vi "Visa Write Trigger.vi"() -> ()   [LabVIEW 2022 SP3]
uses:
  <vilib>/Instr/_visa.llb/Select Event Type.ctl
panel:
  in  "2400 CURR LIST":string="20E-6,-20E-6"
  out "Resistance of DUT":dbl[](graph)
  out "Resistance (m-Ohms)":dbl[](array[numeric]) format="%.10f"
  in  "Sample Count To Display":i32=10
  out "Voltage Drop Across DUT":dbl[](graph)
  out "Delta Readings (uV)":ext[](array[numeric]) format="%.12f"
  in  "2400 Trig Count":string="20"
  in  "2182A":T1={"Baud Rate"=9600, "Parity"=0, "Data Bits"=8, "Stop Bits"=10, "Flow Control"=0, "VISA resource name"="NanoVoltMeter2182"} {"Flow Control" items=["None", "XON/XOFF", "RTS/CTS", "XON/XOFF & RTS/CTS", "DTR/DSR", "XON/XOFF & DTR/DSR"]; "Stop Bits" items=["1.0"=10, "1.5"=15, "2.0"=20]; "Data Bits" items=["7"=7, "8"=8]; "Parity" items=["None", "Odd", "Even", "Mark", "Space"]; "Baud Rate" items=["300"=300, "600"=600, "1200"=1200, "2400"=2400, "4800"=4800, "9600"=9600, "19200"=19200]}
  in  "2400":T1={"Baud Rate"=9600, "Parity"=0, "Data Bits"=8, "Stop Bits"=10, "Flow Control"=0, "VISA resource name"="NanoVoltMeter2182"} {"Flow Control" items=["None", "XON/XOFF", "RTS/CTS", "XON/XOFF & RTS/CTS", "DTR/DSR", "XON/XOFF & DTR/DSR"]; "Stop Bits" items=["1.0"=10, "1.5"=15, "2.0"=20]; "Data Bits" items=["7"=7, "8"=8]; "Parity" items=["None", "Odd", "Even", "Mark", "Space"]; "Baud Rate" items=["300"=300, "600"=600, "1200"=1200, "2400"=2400, "4800"=4800, "9600"=9600, "19200"=19200]}
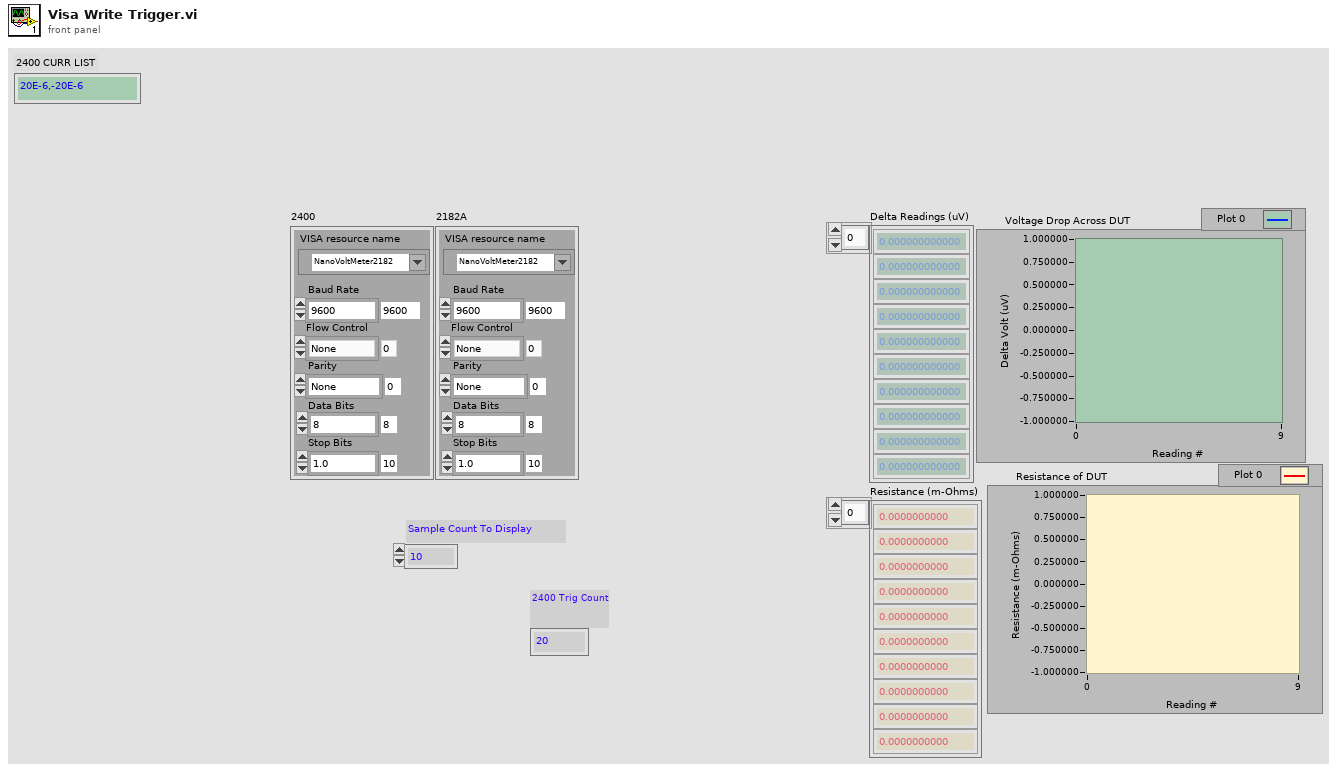
[diagram p1: front panel]
types:
  T1 = cluster{"Baud Rate":u32, "Parity":u16, "Data Bits":u16, "Stop Bits":u16, "Flow Control":u16, "VISA resource name":refnum<visa-resource-name>}
  T2 = typedef "Select Event Type.ctl" = u32
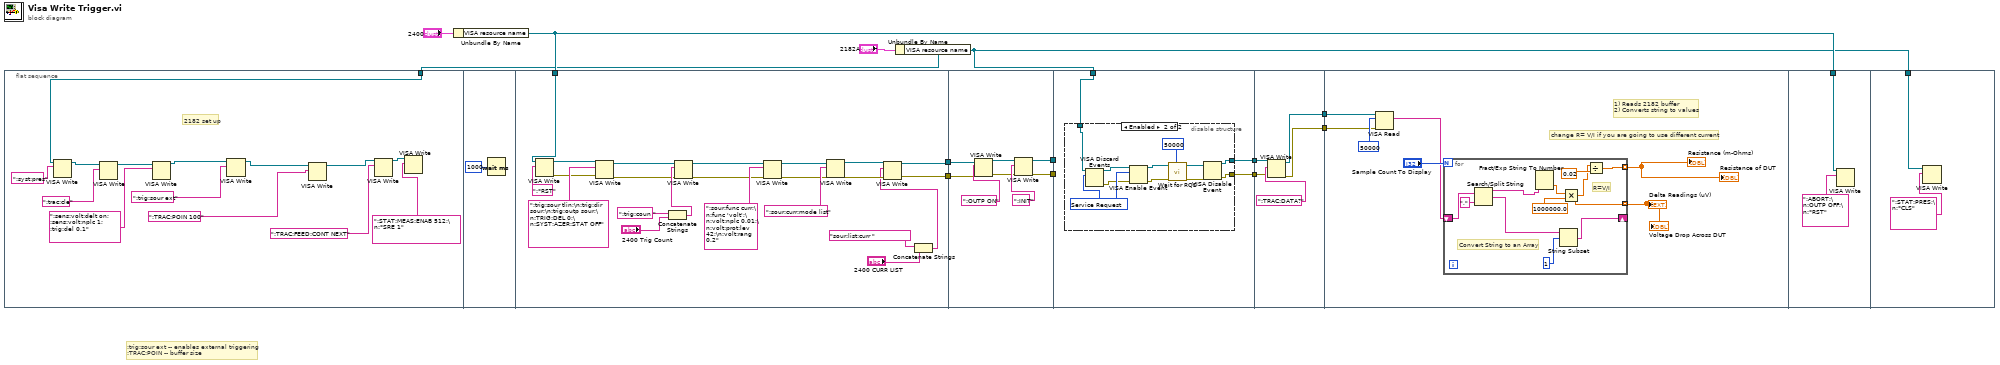
[diagram p0: block diagram]
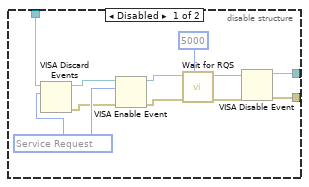
[diagram p2: hidden frame]
diagram:
  # ":trig:sour ext -- enables external triggering\n:TRAC:POIN -- buffer size"
  n1 = flat-sequence {
    tunnel: w2 -> [w25]
    tunnel: w6 -> [w50]
    tunnel: [w33] -> w11
    tunnel: [w32] -> w1
    tunnel: w11 -> [w58]
    tunnel: [w52] -> w10
    tunnel: [w51] -> w9
    tunnel: w1 -> [w54]
    tunnel: w10 -> [_]
    tunnel: w9 -> [_]
    tunnel: w2 -> [w61]
    tunnel: [w60] -> w5
    tunnel: [w59] -> w4
    tunnel: [w87] -> w8
    tunnel: [w86] -> w7
    tunnel: w5 -> [w85]
    tunnel: w4 -> [w84]
    tunnel: w8 -> [w90]
    tunnel: w7 -> [w89]
    tunnel: w6 -> [w108]
    tunnel: w2 -> [w110]
    frame #0 {
      # "2182 set up"
      n2 = VISA Write(VISA resource name=w25, write buffer=":syst:pres") -> (VISA resource name out=w24:refnum<visa-resource-name>)  [unwired: 1 in, 2 out]
      n3 = VISA Write(VISA resource name=w24, write buffer=":trac:cle") -> (VISA resource name out=w23:refnum<visa-resource-name>)  [unwired: 1 in, 2 out]
      n4 = VISA Write(VISA resource name=w23, write buffer=":sens:volt:delt on; :sens:volt:nplc 1; :trig:del 0.1") -> (VISA resource name out=w22:refnum<visa-resource-name>)  [unwired: 1 in, 2 out]
      n5 = VISA Write(VISA resource name=w22, write buffer=":trig:sour ext") -> (VISA resource name out=w21:refnum<visa-resource-name>)  [unwired: 1 in, 2 out]
      n6 = VISA Write(VISA resource name=w21, write buffer=":TRAC:POIN 100") -> (VISA resource name out=w20:refnum<visa-resource-name>)  [unwired: 1 in, 2 out]
      n7 = VISA Write(VISA resource name=w20, write buffer=":TRAC:FEED:CONT NEXT") -> (VISA resource name out=w19:refnum<visa-resource-name>)  [unwired: 1 in, 2 out]
      n8 = VISA Write(VISA resource name=w19, write buffer=":STAT:MEAS:ENAB 512;\n:*SRE 1") -> ()  [unwired: 1 in, 3 out]
    }
    frame #1 {
      n9 = Wait (ms)(milliseconds to wait=u32 1000) -> ()  [unwired: 1 out]
    }
    frame #2 {
      n10 = VISA Write(VISA resource name=w50, write buffer=":*RST") -> (VISA resource name out=w48:refnum<visa-resource-name>, error out=w38:errorcluster)  [unwired: 1 in, 1 out]
      n11 = VISA Write(VISA resource name=w48, write buffer=":trig:sour tlin;\n:trig:dir sour;\n:trig:outp sour;\n:TRIG:DEL 0;\n:SYST:AZER:STAT OFF", error in (no error)=w38) -> (VISA resource name out=w47:refnum<visa-resource-name>, error out=w37:errorcluster)  [unwired: 1 out]
      n12 = Concatenate Strings(":trig:coun ", "2400 Trig Count") -> (w41:string)
      n13 = VISA Write(VISA resource name=w47, write buffer=w41, error in (no error)=w37) -> (VISA resource name out=w46:refnum<visa-resource-name>, error out=w36:errorcluster)  [unwired: 1 out]
      n14 = VISA Write(VISA resource name=w46, write buffer=":sour:func curr;\n:func 'volt';\n:volt:nplc 0.01;\n:volt:prot:lev 42;\n:volt:rang 0.2", error in (no error)=w36) -> (VISA resource name out=w45:refnum<visa-resource-name>, error out=w35:errorcluster)  [unwired: 1 out]
      n15 = VISA Write(VISA resource name=w45, write buffer=":sour:curr:mode list", error in (no error)=w35) -> (VISA resource name out=w34:refnum<visa-resource-name>, error out=w31:errorcluster)  [unwired: 1 out]
      n16 = Concatenate Strings("sour:list:curr ", "2400 CURR LIST") -> (w28:string)
      n17 = VISA Write(VISA resource name=w34, write buffer=w28, error in (no error)=w31) -> (VISA resource name out=w33:refnum<visa-resource-name>, error out=w32:errorcluster)  [unwired: 1 out]
    }
    frame #3 {
      n18 = VISA Write(VISA resource name=w58, write buffer=":OUTP ON", error in (no error)=w54) -> (VISA resource name out=w57:refnum<visa-resource-name>, error out=w53:errorcluster)  [unwired: 1 out]
      n19 = VISA Write(VISA resource name=w57, write buffer=":INIT", error in (no error)=w53) -> (VISA resource name out=w52:refnum<visa-resource-name>, error out=w51:errorcluster)  [unwired: 1 out]
    }
    frame #4 {
      n20 = disable-structure shown="Enabled" {
        disable-tunnel: w61 -> [w71 w75]
        disable-tunnel: [w64 w74] -> w60
        disable-tunnel: [w62 w73] -> w59
        frame Disabled {
          w68 = T2 1073684491 items=["Service Request"=1073684491, "Trigger"=3221168138, "Clear"=1073684493, "VXI Signal"=1073684512, "VXI/VME Interrupt"=3221168161, "VXI/VME Sysfail"=1073684509, "VXI/VME Sysreset"=1073684510, "GPIB CIC"=1073684498, "GPIB Talk"=1073684499, "GPIB Listen"=1073684500, "PXI Interrupt"=1073684514, "Serial Break"=1073684515, "Serial TermChar"=1073684516, "Serial CTS"=1073684521, "Serial DSR"=1073684522, "Serial DCD"=1073684524, "Serial RI"=1073684526, "Serial Character"=1073684533, "USB Interrupt"=1073684535, "All Enabled"=1073709055] ("Event Type")
          n21 = VISA Discard Events(10:w68, 11:w71) -> (0:w66:errorcluster, 3:w70:refnum<visa-resource-name>)  [unwired: 2 in]
          n22 = VISA Enable Event(8:w66, 10:w68, 11:w70) -> (0:w67:errorcluster, 3:w69:refnum<visa-resource-name>)  [unwired: 1 in]
          n23 = call <vilib>:"Wait for RQS.vi"("timeout (25000 ms)"=u32 5000, "error in (no error)"=w67, "VISA resource name"=w69) -> ("error out"=w63:errorcluster, "VISA resource name out"=w65:refnum<visa-resource-name>)  [unwired: 6 in, 1 out]
          n24 = VISA Disable Event(8:w63, 11:w65) -> (0:w62:errorcluster, 3:w64:refnum<visa-resource-name>)  [unwired: 2 in]
        }
        frame Enabled {
          w80 = T2 1073684491 items=["Service Request"=1073684491, "Trigger"=3221168138, "Clear"=1073684493, "VXI Signal"=1073684512, "VXI/VME Interrupt"=3221168161, "VXI/VME Sysfail"=1073684509, "VXI/VME Sysreset"=1073684510, "GPIB CIC"=1073684498, "GPIB Talk"=1073684499, "GPIB Listen"=1073684500, "PXI Interrupt"=1073684514, "Serial Break"=1073684515, "Serial TermChar"=1073684516, "Serial CTS"=1073684521, "Serial DSR"=1073684522, "Serial DCD"=1073684524, "Serial RI"=1073684526, "Serial Character"=1073684533, "USB Interrupt"=1073684535, "All Enabled"=1073709055] ("Event Type")
          n25 = VISA Discard Events(10:w80, 11:w75) -> (0:w78:errorcluster, 3:w82:refnum<visa-resource-name>)  [unwired: 2 in]
          n26 = VISA Enable Event(8:w78, 10:w80, 11:w82) -> (0:w79:errorcluster, 3:w81:refnum<visa-resource-name>)  [unwired: 1 in]
          n27 = call <vilib>:"Wait for RQS.vi"("timeout (25000 ms)"=u32 50000, "error in (no error)"=w79, "VISA resource name"=w81) -> ("error out"=w76:errorcluster, "VISA resource name out"=w77:refnum<visa-resource-name>)  [unwired: 6 in, 1 out]
          n28 = VISA Disable Event(8:w76, 11:w77) -> (0:w73:errorcluster, 3:w74:refnum<visa-resource-name>)  [unwired: 2 in]
        }
      }
    }
    frame #5 {
      n29 = VISA Write(VISA resource name=w85, write buffer=":TRAC:DATA?", error in (no error)=w84) -> (VISA resource name out=w87:refnum<visa-resource-name>, error out=w86:errorcluster)  [unwired: 1 out]
    }
    frame #6 {
      # "1) Reads 2182 buffer\n2) Converts string to values"
      # "change R= V/I if you are going to use different current"
      n30 = VISA Read(VISA resource name=w90, byte count=50000, error in (no error)=w89) -> (read buffer=w91:string)  [unwired: 3 out]
      n31 = for {
        N: "Sample Count To Display" -> [_]
        tunnel: [w97] -> w94 mode=indexing
        shift-right: [w102] -> _
        shift-left: w91 -> [w103]
        tunnel: [w99] -> w93 mode=indexing
        # "R=V/I"
        # "Convert String to an Array"
        n32 = Search/Split String(string=w103, search string/char (-)=",") -> (substring before match=w105:string, match + rest of string=w104:string)  [unwired: 1 in, 1 out]
        n33 = Fract/Exp String To Number(string=w105) -> (number=w96:dbl)  [unwired: 3 in, 1 out]
        n34 = String Subset(string=w104, offset (0)=1) -> (substring=w102:string)  [unwired: 1 in]
        n35 = Multiply(x=w96, y=1000000.0) -> (x*y=w97:dbl)
        n36 = Divide(x=w97, y=0.02 ("x")) -> (x/y=w99:dbl)
      }
      "Delta Readings (uV)" <- w94
      "Voltage Drop Across DUT" <- w94
      "Resistance (m-Ohms)" <- w93
      "Resistance of DUT" <- w93
    }
    frame #7 {
      n37 = VISA Write(VISA resource name=w108, write buffer=":ABORT;\n:OUTP OFF;\n:*RST" ("data")) -> ()  [unwired: 1 in, 3 out]
    }
    frame #8 {
      n38 = VISA Write(VISA resource name=w110, write buffer=":STAT:PRES;\n:*CLS" ("data")) -> ()  [unwired: 1 in, 3 out]
    }
  }
  n39 = Unbundle By Name("2400") -> ("VISA resource name"=w6:refnum<visa-resource-name>)
  n40 = Unbundle By Name("2182A") -> ("VISA resource name"=w2:refnum<visa-resource-name>)
